vi "SessionManagementService ReserveSessions.vi"(6 "contextId":T1, 8 "error in":errorcluster, 9 "timeout (ms)":i32=-1, 10 "Request Data":T9, 11 "gRPC ID":T1) -> (0 "error out":errorcluster, 2 "Response Data":T2, 3 "gRPC ID out":T1)   [LabVIEW 2020, in "Measurement Plugin Session Management Client.lvlib"]
uses:
  Measurement Plugin Session Management Client.lvlib
  <vilib>/gRPC/LabVIEW gRPC Library/Shared/grpcId.ctl
  RPC Messages/ni_measurementlink_sessionmanagement_v1_ReserveSessionsRequest.ctl
  RPC Messages/ni_measurementlink_PinMapContext.ctl
  RPC Messages/ni_measurementlink_sessionmanagement_v1_ReserveSessionsResponse.ctl
  RPC Messages/ni_measurementlink_sessionmanagement_v1_SessionInformation.ctl
  RPC Messages/nidevice_grpc_Session.ctl
  RPC Messages/ni_measurementlink_sessionmanagement_v1_ChannelMapping.ctl
  RPC Messages/ni_measurementlink_sessionmanagement_v1_MultiplexerSessionInformation.ctl
  RPC Messages/ni_measurementlink_sessionmanagement_v1_ReserveSessionsResponse_GroupMappingsEntry.ctl
  RPC Messages/ni_measurementlink_sessionmanagement_v1_ResolvedPinsOrRelays.ctl
  RPC Messages/ni_measurementlink_sessionmanagement_v1_ReserveSessionsResponse_Flat.ctl
  RPC Messages/ni_measurementlink_sessionmanagement_v1_SessionInformation_Flat.ctl
  RPC Messages/nidevice_grpc_Session_Flat.ctl
  RPC Messages/ni_measurementlink_sessionmanagement_v1_ChannelMapping_Flat.ctl
  RPC Messages/ni_measurementlink_sessionmanagement_v1_MultiplexerSessionInformation_Flat.ctl
  RPC Messages/ni_measurementlink_sessionmanagement_v1_ReserveSessionsResponse_GroupMappingsEntry_Flat.ctl
  RPC Messages/ni_measurementlink_sessionmanagement_v1_ResolvedPinsOrRelays_Flat.ctl
  14035477-4c25-4107-8ed5-d0c4ef420ce5.vi
  RPC Messages/RichToFlatni_measurementlink_PinMapContext.vi
  <vilib>/gRPC/LabVIEW gRPC Library/Shared/TranslateGrpcError.vi
  <vilib>/gRPC/LabVIEW gRPC Library/Shared/Wait On Occurence.vi
  RPC Messages/FlatToRichni_measurementlink_sessionmanagement_v1_SessionInformation.vi
  RPC Messages/FlatToRichni_measurementlink_sessionmanagement_v1_MultiplexerSessionInformation.vi
  RPC Messages/FlatToRichni_measurementlink_sessionmanagement_v1_ReserveSessionsResponse_GroupMappingsEntry.vi
  RPC Messages/FlatToRichnidevice_grpc_Session.vi
  RPC Messages/FlatToRichni_measurementlink_sessionmanagement_v1_ChannelMapping.vi
  RPC Messages/FlatToRichni_measurementlink_sessionmanagement_v1_ResolvedPinsOrRelays.vi
  <vilib>/gRPC/LabVIEW gRPC Library/Server API/Server/Get Server DLL Path.vi
  <vilib>/Utility/error.llb/Error Cluster From Error Code.vi
  <vilib>/Utility/error.llb/Simple Error Handler.vi
  <vilib>/gRPC/LabVIEW gRPC Library/grpc-lvsupport-release.lvlib
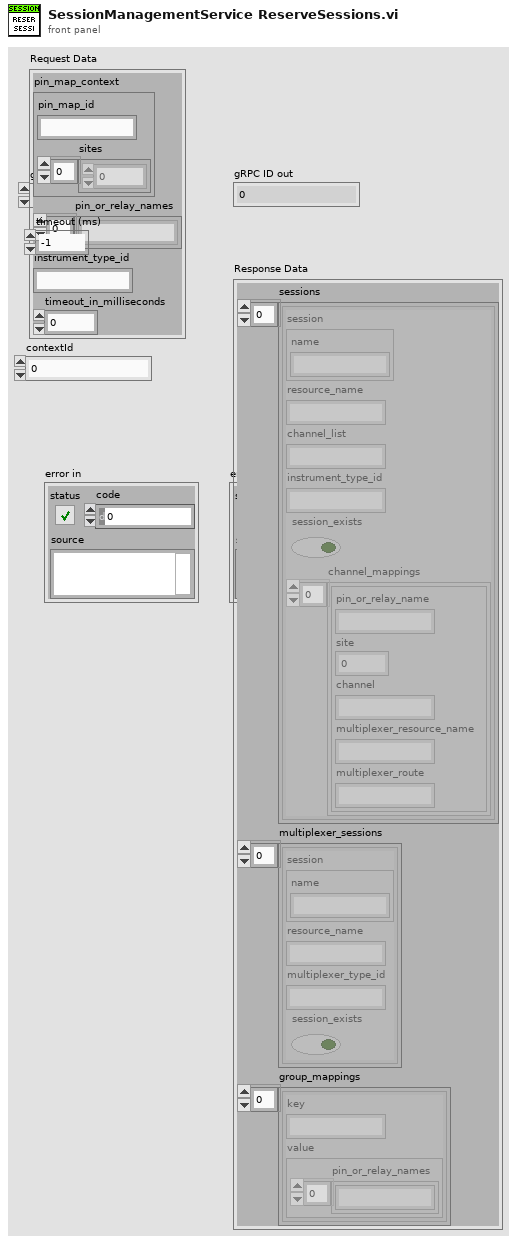
[diagram p1: front panel]
types:
  T1 = typedef "grpc-lvsupport-release.lvlib/grpcId.ctl" = u64
  T2 = typedef "Measurement Plugin Session Management Client.lvlib/ni_measurementlink_sessionmanagement_v1_ReserveSessionsResponse.ctl" = cluster{"sessions":T3[], "multiplexer_sessions":T6[], "group_mappings":T7[]}
  T3 = typedef "Measurement Plugin Session Management Client.lvlib/ni_measurementlink_sessionmanagement_v1_SessionInformation.ctl" = cluster{"session":T4, "resource_name":string, "channel_list":string, "instrument_type_id":string, "session_exists":bool, "channel_mappings":T5[]}
  T4 = typedef "Measurement Plugin Session Management Client.lvlib/nidevice_grpc_Session.ctl" = cluster{"name":string}
  T5 = typedef "Measurement Plugin Session Management Client.lvlib/ni_measurementlink_sessionmanagement_v1_ChannelMapping.ctl" = cluster{"pin_or_relay_name":string, "site":i32, "channel":string, "multiplexer_resource_name":string, "multiplexer_route":string}
  T6 = typedef "Measurement Plugin Session Management Client.lvlib/ni_measurementlink_sessionmanagement_v1_MultiplexerSessionInformation.ctl" = cluster{"session":T4, "resource_name":string, "multiplexer_type_id":string, "session_exists":bool}
  T7 = typedef "Measurement Plugin Session Management Client.lvlib/ni_measurementlink_sessionmanagement_v1_ReserveSessionsResponse_GroupMappingsEntry.ctl" = cluster{"key":string, "value":T8}
  T8 = typedef "Measurement Plugin Session Management Client.lvlib/ni_measurementlink_sessionmanagement_v1_ResolvedPinsOrRelays.ctl" = cluster{"pin_or_relay_names":string[]}
  T9 = typedef "Measurement Plugin Session Management Client.lvlib/ni_measurementlink_sessionmanagement_v1_ReserveSessionsRequest.ctl" = cluster{"pin_map_context":T10, "pin_or_relay_names":string[], "instrument_type_id":string, "timeout_in_milliseconds":i32}
  T10 = typedef "Measurement Plugin Session Management Client.lvlib/ni_measurementlink_PinMapContext.ctl" = cluster{"pin_map_id":string, "sites":i32[]}
  T11 = typedef "Measurement Plugin Session Management Client.lvlib/ni_measurementlink_sessionmanagement_v1_ReserveSessionsResponse_Flat.ctl" = cluster{"sessions":T12[], "multiplexer_sessions":T15[], "group_mappings":T16[]}
  T12 = typedef "Measurement Plugin Session Management Client.lvlib/ni_measurementlink_sessionmanagement_v1_SessionInformation_Flat.ctl" = cluster{"session":T13, "resource_name":string, "channel_list":string, "instrument_type_id":string, "session_exists":bool, "channel_mappings":T14[]}
  T13 = typedef "Measurement Plugin Session Management Client.lvlib/nidevice_grpc_Session_Flat.ctl" = cluster{"name":string}
  T14 = typedef "Measurement Plugin Session Management Client.lvlib/ni_measurementlink_sessionmanagement_v1_ChannelMapping_Flat.ctl" = cluster{"pin_or_relay_name":string, "site":i32, "channel":string, "multiplexer_resource_name":string, "multiplexer_route":string}
  T15 = typedef "Measurement Plugin Session Management Client.lvlib/ni_measurementlink_sessionmanagement_v1_MultiplexerSessionInformation_Flat.ctl" = cluster{"session":T13, "resource_name":string, "multiplexer_type_id":string, "session_exists":bool}
  T16 = typedef "Measurement Plugin Session Management Client.lvlib/ni_measurementlink_sessionmanagement_v1_ReserveSessionsResponse_GroupMappingsEntry_Flat.ctl" = cluster{"key":string, "value":T17}
  T17 = typedef "Measurement Plugin Session Management Client.lvlib/ni_measurementlink_sessionmanagement_v1_ResolvedPinsOrRelays_Flat.ctl" = cluster{"pin_or_relay_names":string[]}
  T18 = typedef "Measurement Plugin Session Management Client.lvlib/ni_measurementlink_sessionmanagement_v1_ReserveSessionsRequest_Flat.ctl" = cluster{"pin_map_context":T19, "pin_or_relay_names":string[], "instrument_type_id":string, "timeout_in_milliseconds":i32}
  T19 = typedef "Measurement Plugin Session Management Client.lvlib/ni_measurementlink_PinMapContext_Flat.ctl" = cluster{"pin_map_id":string, "sites":i32[]}
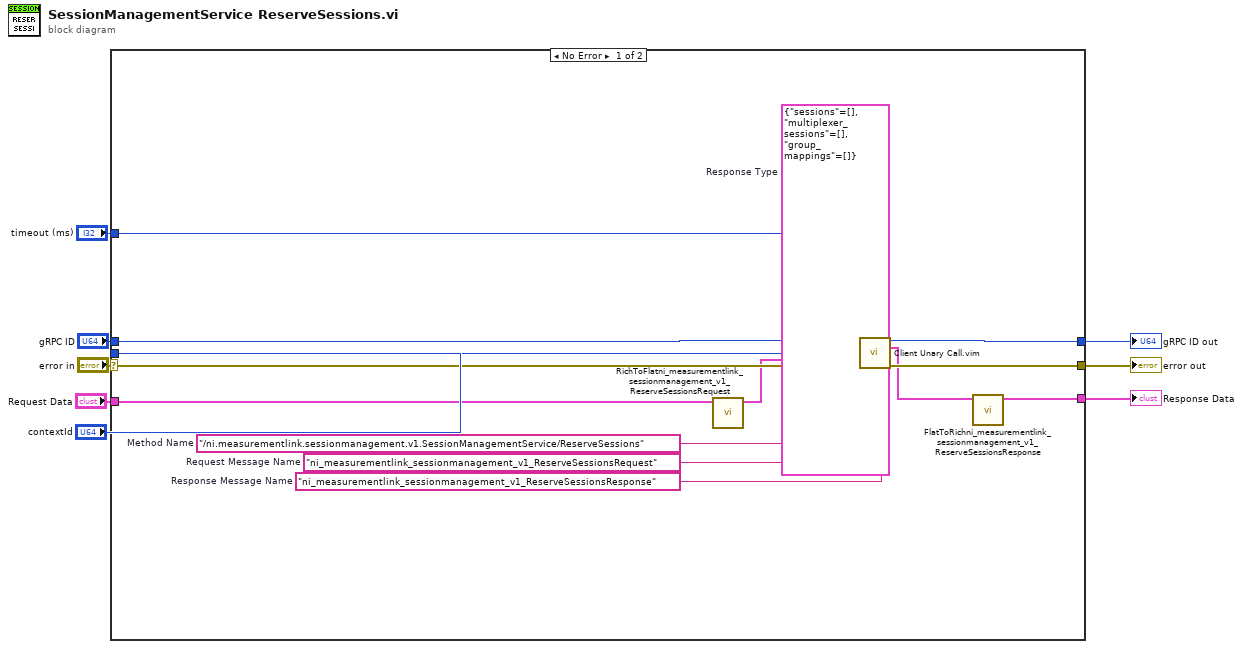
[diagram p0: block diagram]
diagram:
  n1 = case shown="No Error" "error in" {
    selector: "error in" -> [w18 w23]
    tunnel: [w17 w23] -> w7
    tunnel: "gRPC ID" -> [w16 w24]
    tunnel: [w15 w24] -> w5
    tunnel: "Request Data" -> [w12 _]
    tunnel: [w9 _] -> w3
    tunnel: "timeout (ms)" -> [w14 _]
    tunnel: "contextId" -> [w13 _]
    frame No Error {
      w19 = "ni_measurementlink_sessionmanagement_v1_ReserveSessionsResponse"  # Response Message Name
      w20 = "ni_measurementlink_sessionmanagement_v1_ReserveSessionsRequest"  # Request Message Name
      w21 = T11 {"sessions"=[], "multiplexer_sessions"=[], "group_mappings"=[]}  # Response Type
      w22 = "/ni.measurementlink.sessionmanagement.v1.SessionManagementService/ReserveSessions"  # Method Name
      n2 = call "RichToFlatni_measurementlink_sessionmanagement_v1_ReserveSessionsRequest.vi"("InputCluster"=w12) -> ("OutputCluster"=w11:T18)  [unwired: 10 in]
      n3 = call "Client Unary Call.vim"("ClientID in"=w16, "Response Type"=w21, "timeout (ms)"=w14, "Method Name"=w22, "contextId"=w13, "Request Data"=w11, "error in"=w18, "Request Message Name"=w20, "Response Message Name"=w19) -> ("ClientID out"=w15:u64, "Response Data"=w10:T11, "error out"=w17:errorcluster)  [unwired: 4 in]
      n4 = call "FlatToRichni_measurementlink_sessionmanagement_v1_ReserveSessionsResponse.vi"("InputCluster"=w10) -> ("OutputCluster"=w9:T2)  [unwired: 10 in]
    }
    frame Error {
    }
  }
  "error out" <- w7
  "gRPC ID out" <- w5
  "Response Data" <- w3
